vi "main.vi"() -> ()   [LabVIEW 2017]
uses:
  <vilib>/Utility/miscctls.llb/LVRectTypeDef.ctl
  <vilib>/Utility/file.llb/Write Delimited Spreadsheet (string).vi
  <vilib>/Utility/file.llb/Read Delimited Spreadsheet (string).vi
panel:
  in  "Time Unit":u16(ring) caption="Relative Time Units" items=["SMART", "Seconds", "Minutes", "Hours", "All"]
  in  "OK Button":bool
  out "String":string
  in  "Select Folder":path
  # "1. Place all spectra you wish to combine into a new folder. Make sure there are no other files in that folder.\n2. Click the folder icon and select your created folder.\n3. Choose what units to use for relative time, then press go.\n4. Save the compiled spreadsheet. Call it whatever you'd like, and put \".csv\" at the end."
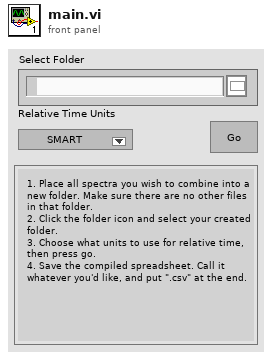
[diagram p1: front panel]
types:
  T1 = typedef "LVRectTypeDef.ctl" = cluster{"Left":i16, "Top":i16, "Right":i16, "Bottom":i16}
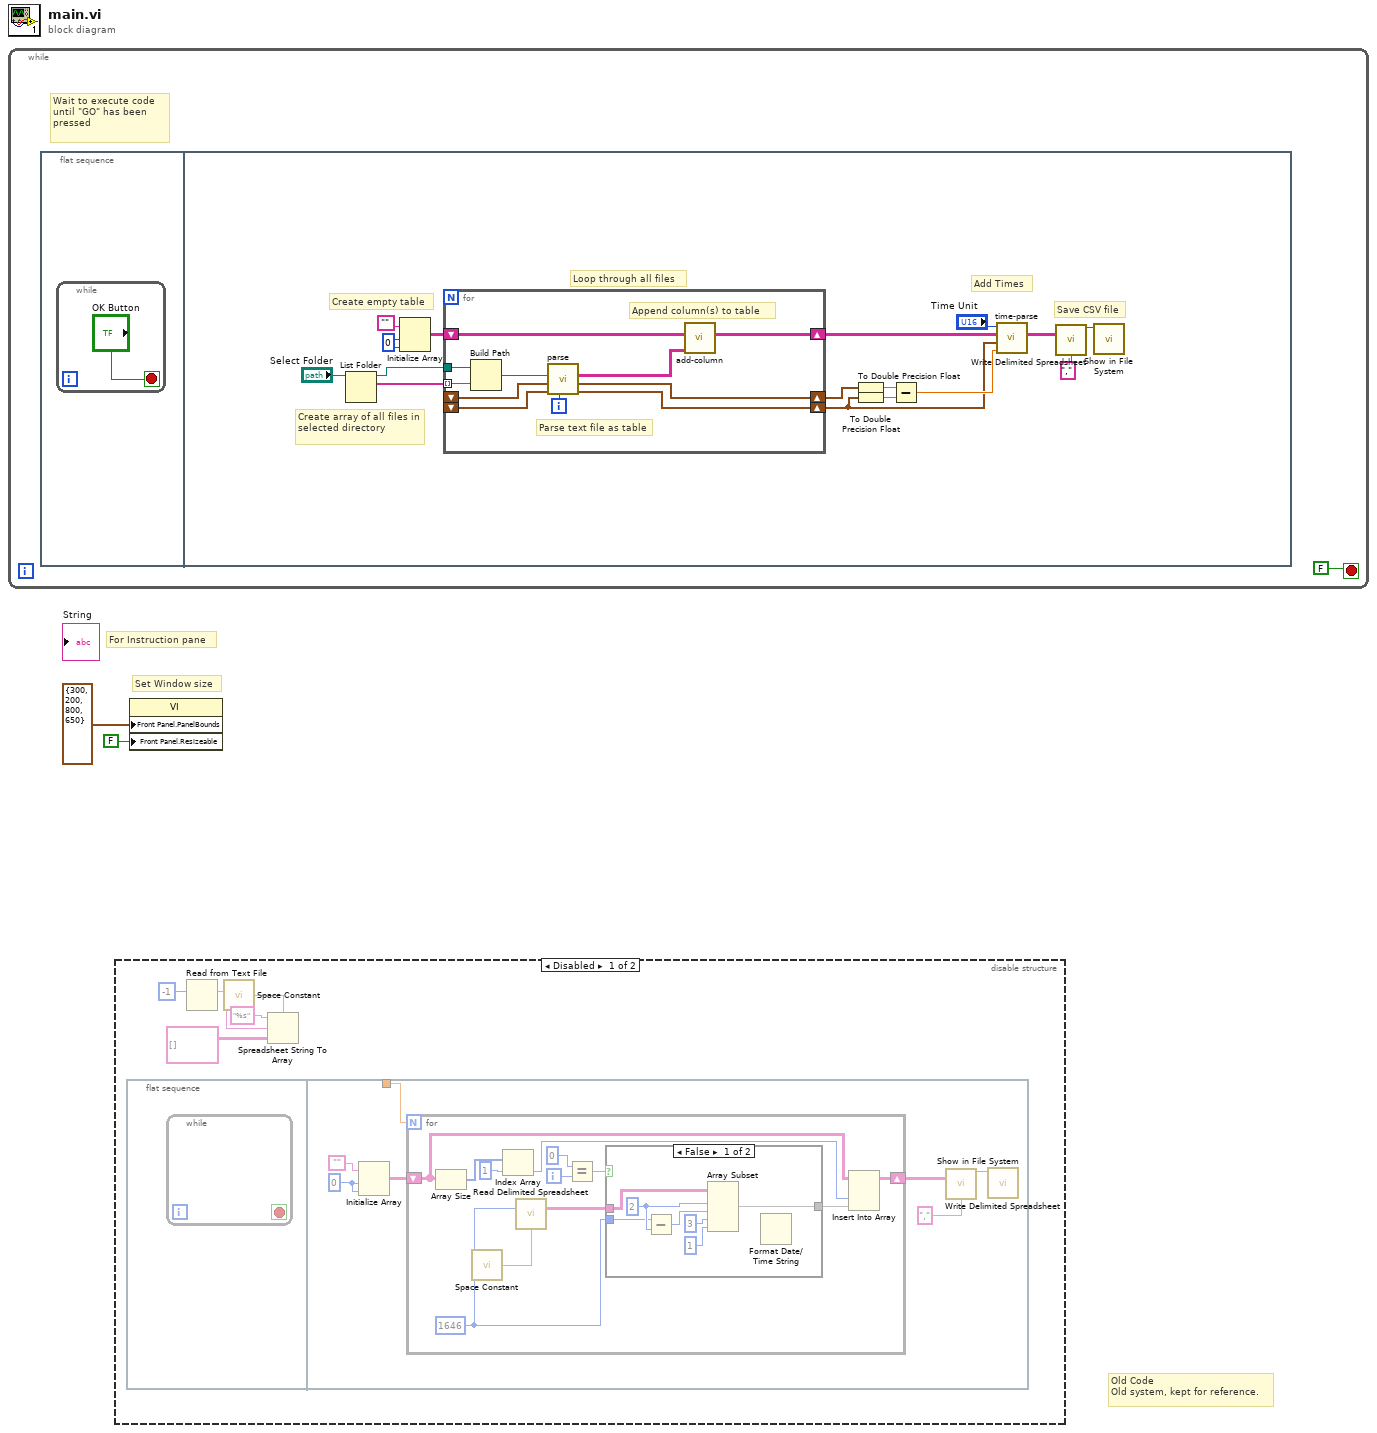
[diagram p0: block diagram]
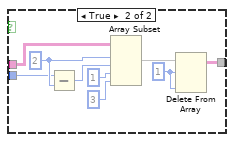
[diagram p2: hidden frame]
diagram:
  # "Set Window size"
  # "For Instruction pane"
  # "Old Code\nOld system, kept for reference."
  n1 = while {
    stop <- FALSE stop-if-true
    # "Wait to execute code until \"GO\" has been pressed"
    n2 = flat-sequence {
      frame #0 {
        n3 = while {
          stop <- "OK Button" stop-if-true
        }
      }
      frame #1 {
        w16 = 0 ("dimension size")
        # "Add Times"
        # "Save CSV file"
        # "Loop through all files"
        # "Create empty table"
        # "Create array of all files in selected directory"
        n4 = List Folder(path="Select Folder") -> (path out=w19:path, filenames=w20:string[])  [unwired: 3 in, 2 out]
        n5 = Initialize Array("", w16, w16) -> (w18:string[][])
        n6 = for {
          shift-right: [w27] -> w8
          shift-left: w18 -> [w28]
          tunnel: w19 -> [w31]
          tunnel: w20 -> [w21] mode=indexing
          shift-right: [w22] -> w5
          shift-left: _ -> [w24]
          shift-right: [w23] -> w7
          shift-left: _ -> [w25]
          i -> [w26]
          # "Append column(s) to table"
          # "Parse text file as table"
          n7 = Build Path(base path=w31, name or relative path=w21) -> (appended path=w30:path)
          n8 = call "parse.vi"("iterative"=w26, "ts least"=w24, "ts great"=w25, "file path"=w30) -> ("ts least"=w22:timestamp, "ts great"=w23:timestamp, "Array out"=w29:string[][])  [unwired: 4 in]
          n9 = call "add-column.vi"("New Column(s)"=w29, "Array In"=w28) -> ("Array Out"=w27:string[][])  [unwired: 9 in]
        }
        n10 = To Double Precision Float(number=w7) -> (double precision float=w12:dbl)
        n11 = To Double Precision Float(number=w5) -> (double precision float=w11:dbl)
        n12 = Subtract(x=w12, y=w11) -> (x-y=w10:dbl)
        n13 = call "time-parse.vi"("greatest ts diff"=w10, "ts least"=w5, "Array in"=w8, "type"="Time Unit") -> ("Array out"=w9:string[][])  [unwired: 7 in]
        n14 = call-poly <vilib>:"Write Delimited Spreadsheet.vi"("2D data"=w9, "delimiter (\\t)"=",") -> ("new file path (Not A Path if cancelled)"=w14:path)  [unwired: 12 in, 1 out]
        n15 = call <vilib>:"Show in File System.vi"("file or directory path"=w14) -> ()  [unwired: 10 in, 1 out]
      }
    }
  }
  n16 = disable-structure shown="Disabled" {
    frame Disabled {
      n17 = flat-sequence {
        tunnel: [w44] -> w37
        frame #0 {
          n18 = while {
            stop <- _ stop-if-true
          }
        }
        frame #1 {
          w38 = 0 ("dimension size")
          n19 = Initialize Array("", w38, w38) -> (w43:string[][])
          n20 = for {
            N: w44 -> [_]
            shift-right: [w50] -> w42
            shift-left: w43 -> [w48]
            i -> [w55]
            w52 = 1646
            n21 = Array Size(array=w48) -> (size(s)=w47:i32[])
            n22 = call <vilib>:"Space Constant.vi"() -> ("String"=w53:string)
            n23 = Index Array(array=w47, index=1) -> (element=w45:i32)
            n24 = call-poly <vilib>:"Read Delimited Spreadsheet.vi"("number of rows (all:-1)"=w52, "delimiter (\\t)"=w53) -> ("all rows"=w51:string[][])  [unwired: 8 in, 5 out]
            n25 = Equal?(x=0, y=w55) -> (x = y?=w56:bool)
            n26 = case shown="False" w56 {
              tunnel: w52 -> [w60 w66]
              tunnel: w51 -> [w63 w65]
              tunnel: [w57 w64] -> w49
              frame False {
                w61 = 2 ("index")
                n27 = Subtract(x=w60, y=w61) -> (x-y=w62:i32)
                n28 = Array Subset(array=w63, index (row)=w61, length (row)=w62, index (col)=3 ("index"), length (col)=1 ("length")) -> (w57:string[][])
                n29 = Format Date/Time String() -> ()  [unwired: 3 in, 1 out]
              }
              frame True {
                w70 = 1
                w69 = 2
                n30 = Subtract(x=w66, y=w69) -> (x-y=w72:i32)
                n31 = Array Subset(array=w65, index (row)=w69, length (row)=w72, index (col)=1, length (col)=3) -> (w71:string[][])
                n32 = Delete From Array(array=w71, length=w70, index (col)=w70) -> (array with subset deleted=w64:string[][])  [unwired: 1 in, 1 out]
              }
            }
            n33 = Insert Into Array(array=w48, index (col)=w45, new element=w49) -> (w50:string[][])  [unwired: 1 in]
          }
          n34 = call-poly <vilib>:"Write Delimited Spreadsheet.vi"("2D data"=w42, "delimiter (\\t)"=",") -> ("new file path (Not A Path if cancelled)"=w39:path)  [unwired: 12 in, 1 out]
          n35 = call <vilib>:"Show in File System.vi"("file or directory path"=w39) -> ()  [unwired: 10 in, 1 out]
        }
      }
      n36 = Read from Text File(count=-1) -> (text=w32:string)  [unwired: 3 in, 3 out]
      n37 = call <vilib>:"Space Constant.vi"() -> ("String"=w34:string)
      n38 = Spreadsheet String To Array(delimiter (Tab)=w34, format string="%s", spreadsheet string=w32, array type (2D Dbl)=string[][] [] ("Array")) -> ()  [unwired: 1 out]
    }
    frame Enabled {
    }
  }
  n39 = property class="VI"("Front Panel.PanelBounds"=T1 {"Left"=300, "Top"=200, "Right"=800, "Bottom"=650} ("Front Panel Window:Panel Bounds"), "Front Panel.Resizeable"=FALSE ("Front Panel Window:Resizable")) -> ()  [unwired: 2 in, 2 out]
